vi "GaAs_GaP_wait_SL.vi"(2 "Debug Mode":bool, 3 "Elapsed Time(s)":dbl, 4 "State":enum16{"Edit", "Start", "Run", "End", "Idle"}(ring), 5 "Argument List In":string[](array[string])) -> (0 "Status Out":string, 1 "Argument List Out":string[](array[string]))   [LabVIEW 2011]
panel:
  out "tphase(s)":dbl[](array[numeric])
  out "nstep":dbl
  out "phase":i32
  out "done":bool
  in  "tP wait (s)":dbl
  in  "tP flow (s)":dbl
  in  "P flow (sccm)":dbl
  in  "nPeriods":dbl
  out "tTotal(s)":dbl
  out "tPeriod(s)":dbl
  in  "tAs wait (s)":dbl
  in  "tAs flow (s)":dbl
  in  "As flow (sccm)":dbl
  in  "Cancel":bool
  in  "OK":bool
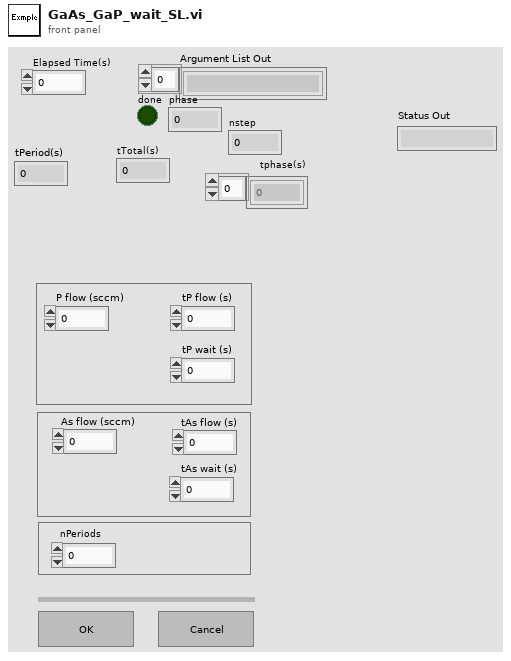
[diagram p1: front panel]
types:
  T1 = enum16{"Discrete", "Continuous", "Instantaneous"}
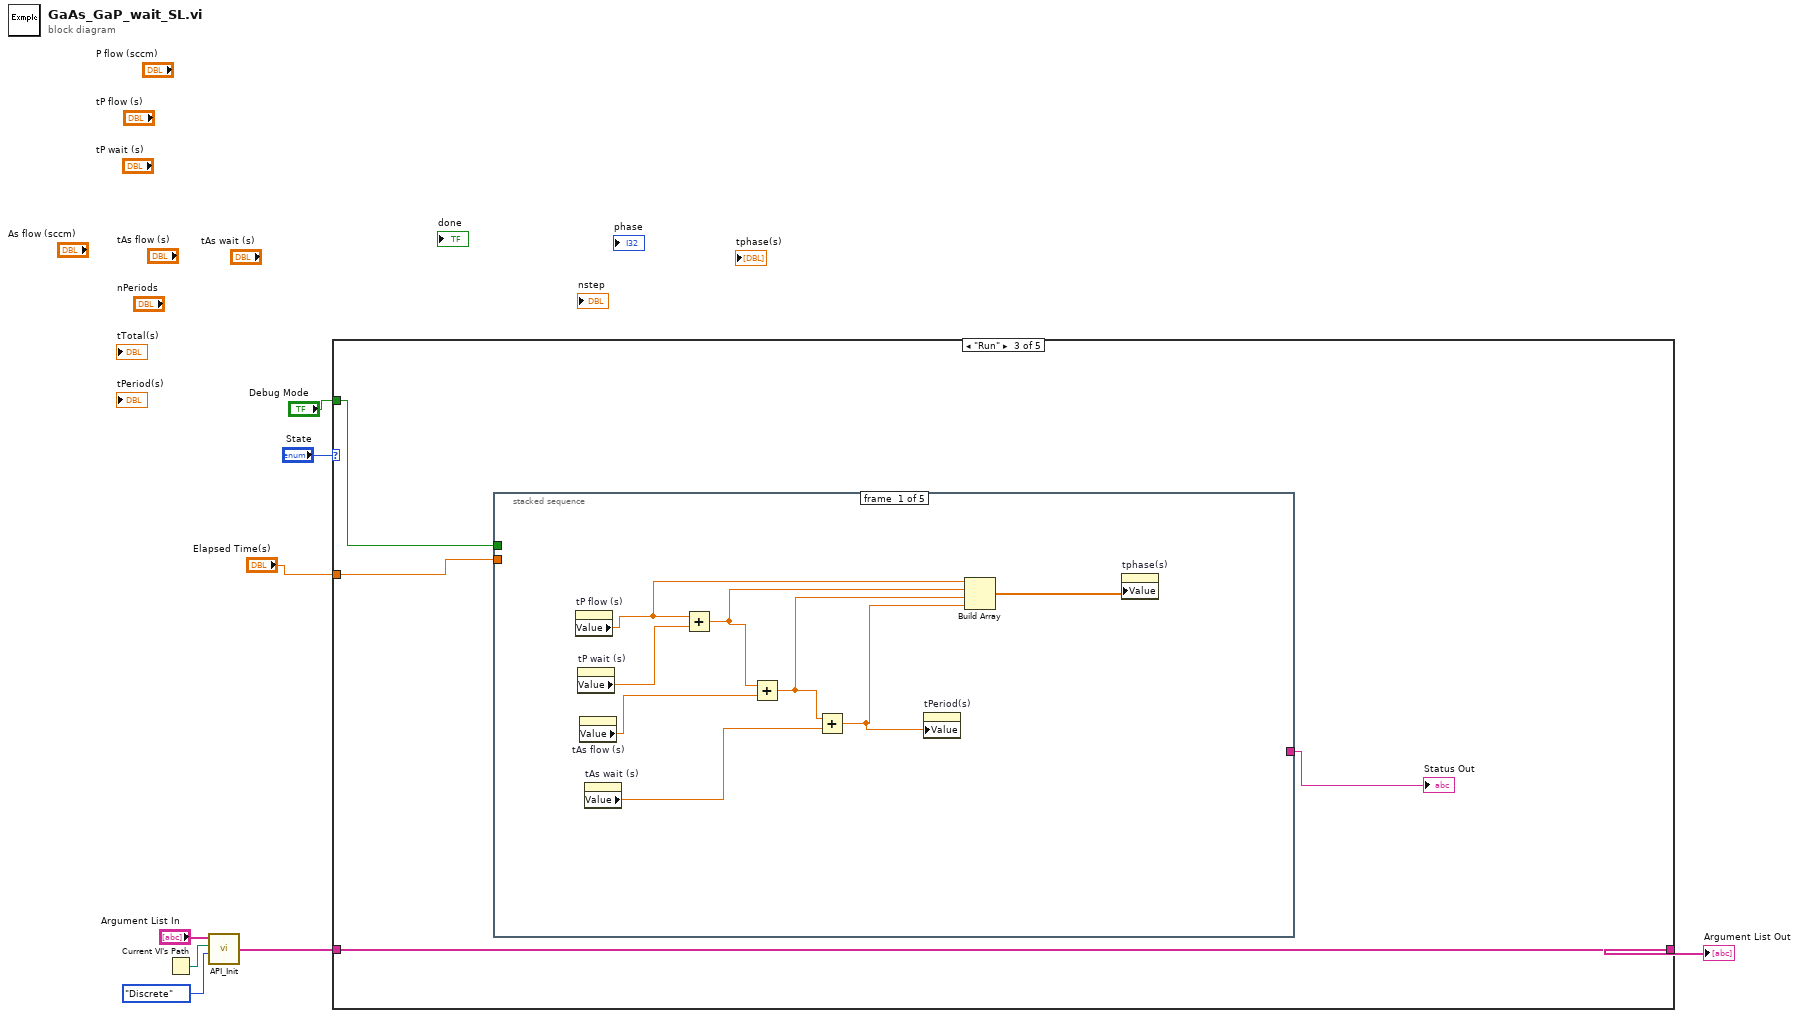
[diagram p0: block diagram]
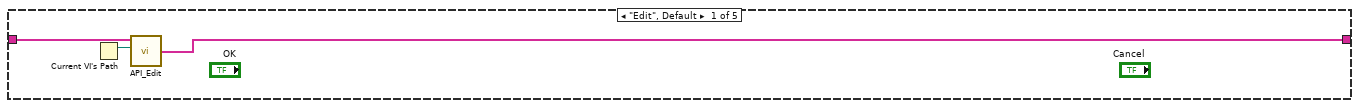
[diagram p2: hidden frame]
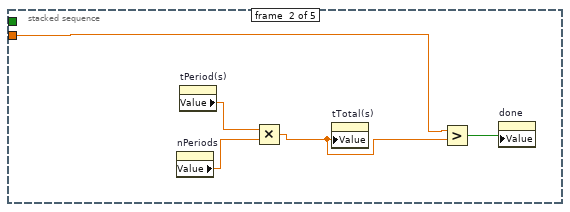
[diagram p4: hidden frame]
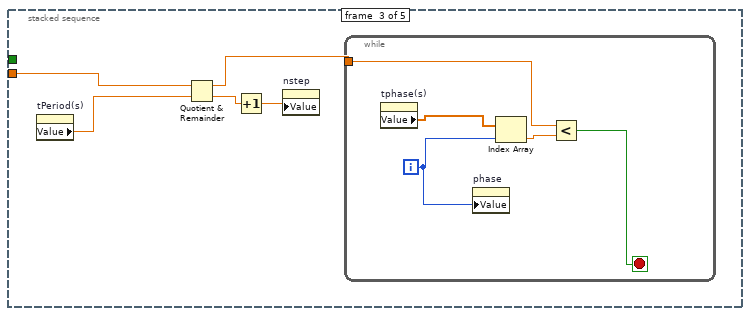
[diagram p5: hidden frame]
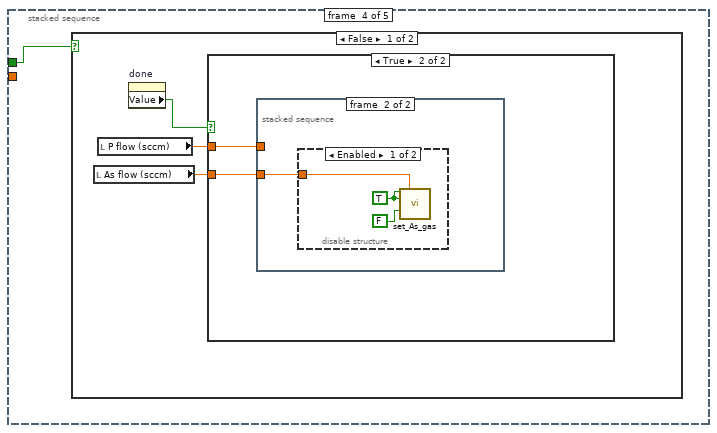
[diagram p6: hidden frame]
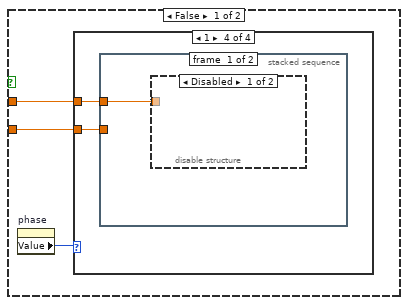
[diagram p7: hidden frame]
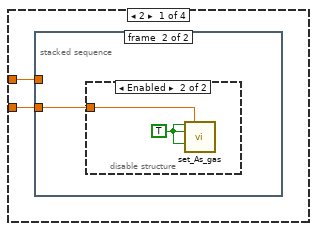
[diagram p8: hidden frame]
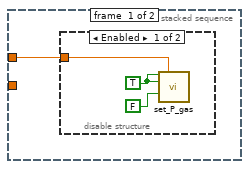
[diagram p9: hidden frame]
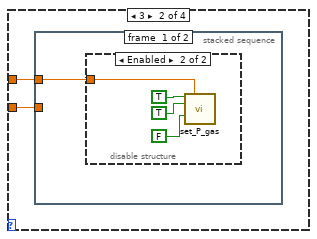
[diagram p12: hidden frame]
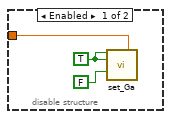
[diagram p15: hidden frame]
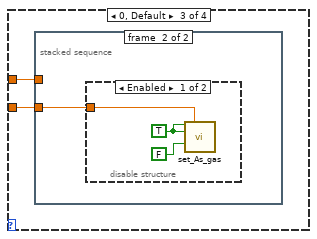
[diagram p16: hidden frame]
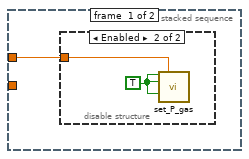
[diagram p17: hidden frame]
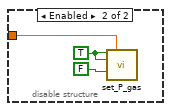
[diagram p20: hidden frame]
diagram:
  n1 = Current VI's Path() -> (path=w5:path)
  n2 = call "API_Init.vi"("API Mode"=T1."Discrete", "VI Path"=w5, "Argument List In"="Argument List In") -> ("Argument List Out"=w6:string[])  [unwired: 1 in]
  n3 = case shown="\"Run\"" "State" {
    tunnel: [w9 w12 w16 w127 w128] -> w2
    tunnel: w6 -> [w11 w12 w16 w127 w128]
    tunnel: "Debug Mode" -> [_ _ w14 _ _]
    tunnel: "Elapsed Time(s)" -> [_ _ w15 _ _]
    frame "Edit", Default {
      n4 = Current VI's Path() -> (path=w10:path)
      n5 = call "API_Edit.vi"("VI Path"=w10, "Argument List In"=w11) -> ("Argument List Out"=w9:string[])  [unwired: 2 in]
    }
    frame "Start" {
    }
    frame "Run" {
      n6 = stacked-sequence {
        tunnel: w15 -> [_ w27 w34 _ _]
        tunnel: w14 -> [_ _ _ w40 _]
        tunnel: [_ _ _ _ w96] -> w13
        frame #0 {
          n7 = property on="tP flow (s)" class="DigNum (strict)"() -> ("Value"=w23:dbl)  [unwired: 2 in, 2 out]
          n8 = property on="tP wait (s)" class="DigNum (strict)"() -> ("Value"=w24:dbl)  [unwired: 2 in, 2 out]
          n9 = property on="tAs flow (s)" class="DigNum (strict)"() -> ("Value"=w21:dbl)  [unwired: 2 in, 2 out]
          n10 = property on="tAs wait (s)" class="DigNum (strict)"() -> ("Value"=w20:dbl)  [unwired: 2 in, 2 out]
          n11 = Add(x=w23, y=w24) -> (x+y=w22:dbl)
          n12 = Add(x=w22, y=w21) -> (x+y=w19:dbl)
          n13 = Add(x=w19, y=w20) -> (x+y=w18:dbl)
          n14 = property on="tPeriod(s)" class="DigNum (strict)"("Value"=w18) -> ()  [unwired: 2 in, 2 out]
          n15 = Build Array(w23, w22, w19, w18) -> (w17:dbl[])
          n16 = property on="tphase(s)" class="Arr (strict)"("Value"=w17) -> ()  [unwired: 2 in, 2 out]
        }
        frame #1 {
          n17 = property on="nPeriods" class="DigNum (strict)"() -> ("Value"=w28:dbl)  [unwired: 2 in, 2 out]
          n18 = property on="tPeriod(s)" class="DigNum (strict)"() -> ("Value"=w29:dbl)  [unwired: 2 in, 2 out]
          n19 = Multiply(x=w29, y=w28) -> (x*y=w26:dbl)
          n20 = property on="tTotal(s)" class="DigNum (strict)"("Value"=w26) -> ()  [unwired: 2 in, 2 out]
          n21 = Greater?(x=w27, y=w26) -> (0:w25:bool)
          n22 = property on="done" class="Bool (strict)"("Value"=w25) -> ()  [unwired: 2 in, 2 out]
        }
        frame #2 {
          n23 = property on="tPeriod(s)" class="DigNum (strict)"() -> ("Value"=w33:dbl)  [unwired: 2 in, 2 out]
          n24 = Quotient & Remainder(x=w34, y=w33) -> (x-y*floor(x/y)=w32:dbl, floor(x/y)=w31:dbl)
          n25 = Increment(x=w31) -> (x+1=w30:dbl)
          n26 = property on="nstep" class="DigNum (strict)"("Value"=w30) -> ()  [unwired: 2 in, 2 out]
          n27 = while {
            tunnel: w32 -> [w38]
            i -> [w36]
            stop <- w35 stop-if-true
            n28 = property on="tphase(s)" class="Arr (strict)"() -> ("Value"=w39:dbl[])  [unwired: 2 in, 2 out]
            n29 = property on="phase" class="DigNum (strict)"("Value"=w36) -> ()  [unwired: 2 in, 2 out]
            n30 = Index Array(array=w39, index=w36) -> (element=w37:dbl)
            n31 = Less?(x=w38, y=w37) -> (x < y?=w35:bool)
          }
        }
        frame #3 {
          n32 = case shown="False" w40 {
            frame False {
              n33 = local read "As flow (sccm)"() -> (w43:dbl)
              n34 = local read "P flow (sccm)"() -> (w42:dbl)
              n35 = property on="done" class="Bool (strict)"() -> ("Value"=w41:bool)  [unwired: 2 in, 2 out]
              n36 = case shown="True" w41 {
                tunnel: w43 -> [w46 w86]
                tunnel: w42 -> [w45 w87]
                frame False {
                  n37 = property on="phase" class="DigNum (strict)"() -> ("Value"=w44:i32)  [unwired: 2 in, 2 out]
                  n38 = case shown="1" w44 {
                    tunnel: w45 -> [w48 w57 w68 w77]
                    tunnel: w46 -> [w47 w56 w67 w76]
                    frame 2 {
                      n39 = stacked-sequence {
                        tunnel: w48 -> [w49 _]
                        tunnel: w47 -> [_ w53]
                        frame #0 {
                          n40 = disable-structure shown="Enabled" {
                            disable-tunnel: w49 -> [w50 _]
                            frame Enabled {
                              w52 = TRUE ("Ga Active")
                              n41 = call "set_P_gas.vi"("P_Gas Active"=w52, "P_Gas Flow"=w50, "P_Gas In"=w52, "P_Gas Run"=FALSE ("Al Run")) -> ()  [unwired: 12 in]
                            }
                            frame Disabled {
                            }
                          }
                        }
                        frame #1 {
                          n42 = disable-structure shown="Enabled" {
                            disable-tunnel: w53 -> [_ w55]
                            frame Disabled {
                            }
                            frame Enabled {
                              w54 = TRUE ("Ga Active")
                              n43 = call "set_As_gas.vi"("As_Gas Active"=w54, "As_Gas Flow"=w55, "As_Gas In"=w54, "As_Gas Run"=w54) -> ()  [unwired: 12 in]
                            }
                          }
                        }
                      }
                    }
                    frame 3 {
                      n44 = stacked-sequence {
                        tunnel: w57 -> [w58 _]
                        tunnel: w56 -> [_ w63]
                        frame #0 {
                          n45 = disable-structure shown="Enabled" {
                            disable-tunnel: w58 -> [_ w59]
                            frame Disabled {
                            }
                            frame Enabled {
                              n46 = call "set_P_gas.vi"("P_Gas Active"=TRUE ("Al Active"), "P_Gas Flow"=w59, "P_Gas In"=TRUE ("Al Bubbler"), "P_Gas Run"=FALSE ("Al Run")) -> ()  [unwired: 12 in]
                            }
                          }
                        }
                        frame #1 {
                          n47 = disable-structure shown="Disabled" {
                            disable-tunnel: w63 -> [w64 _]
                            frame Enabled {
                              w65 = TRUE ("Ga Active")
                              n48 = call "set_Ga.vi"("Ga Active"=w65, "Ga Flow 1"=w64, "Ga Bubbler"=w65, "Ga Run"=FALSE) -> ()  [unwired: 4 in, 8 out]
                            }
                            frame Disabled {
                            }
                          }
                        }
                      }
                    }
                    frame 0, Default {
                      n49 = stacked-sequence {
                        tunnel: w68 -> [w69 _]
                        tunnel: w67 -> [_ w72]
                        frame #0 {
                          n50 = disable-structure shown="Enabled" {
                            disable-tunnel: w69 -> [_ w71]
                            frame Disabled {
                            }
                            frame Enabled {
                              w70 = TRUE ("Al Active")
                              n51 = call "set_P_gas.vi"("P_Gas Active"=w70, "P_Gas Flow"=w71, "P_Gas In"=w70, "P_Gas Run"=w70) -> ()  [unwired: 12 in]
                            }
                          }
                        }
                        frame #1 {
                          n52 = disable-structure shown="Enabled" {
                            disable-tunnel: w72 -> [w73 _]
                            frame Enabled {
                              w74 = TRUE ("Ga Active")
                              n53 = call "set_As_gas.vi"("As_Gas Active"=w74, "As_Gas Flow"=w73, "As_Gas In"=w74, "As_Gas Run"=FALSE ("Ga Run")) -> ()  [unwired: 12 in]
                            }
                            frame Disabled {
                            }
                          }
                        }
                      }
                    }
                    frame 1 {
                      n54 = stacked-sequence {
                        tunnel: w76 -> [_ w82]
                        tunnel: w77 -> [w78 _]
                        frame #0 {
                          n55 = disable-structure shown="Disabled" {
                            disable-tunnel: w78 -> [_ w80]
                            frame Disabled {
                            }
                            frame Enabled {
                              w79 = TRUE ("Al Bubbler")
                              n56 = call "set_P_gas.vi"("P_Gas Active"=w79, "P_Gas Flow"=w80, "P_Gas In"=w79, "P_Gas Run"=FALSE ("Al Run")) -> ()  [unwired: 12 in]
                            }
                          }
                        }
                        frame #1 {
                          n57 = disable-structure shown="Disabled" {
                            disable-tunnel: w82 -> [w83 _]
                            frame Enabled {
                              w84 = TRUE ("Ga Active")
                              n58 = call "set_As_gas.vi"("As_Gas Active"=w84, "As_Gas Flow"=w83, "As_Gas In"=w84, "As_Gas Run"=FALSE ("Ga Run")) -> ()  [unwired: 12 in]
                            }
                            frame Disabled {
                            }
                          }
                        }
                      }
                    }
                  }
                }
                frame True {
                  n59 = stacked-sequence {
                    tunnel: w87 -> [w88 _]
                    tunnel: w86 -> [_ w92]
                    frame #0 {
                      n60 = disable-structure shown="Enabled" {
                        disable-tunnel: w88 -> [_ w91]
                        frame Disabled {
                        }
                        frame Enabled {
                          w90 = TRUE ("Al Active")
                          n61 = call "set_Al.vi"("Aluminum Flow"=w91, "Al Run"=FALSE, "Al Bubbler"=w90, "Al Active"=w90) -> ()  [unwired: 6 in]
                        }
                      }
                    }
                    frame #1 {
                      n62 = disable-structure shown="Enabled" {
                        disable-tunnel: w92 -> [w93 _]
                        frame Enabled {
                          w94 = TRUE ("Ga Active")
                          n63 = call "set_As_gas.vi"("As_Gas Active"=w94, "As_Gas Flow"=w93, "As_Gas In"=w94, "As_Gas Run"=FALSE ("Ga Run")) -> ()  [unwired: 12 in]
                        }
                        frame Disabled {
                        }
                      }
                    }
                  }
                }
              }
            }
            frame True {
            }
          }
        }
        frame #4 {
          n64 = property on="done" class="Bool (strict)"() -> ("Value"=w97:bool)  [unwired: 2 in, 2 out]
          n65 = case shown="True" w97 {
            tunnel: [w98 w126] -> w96
            frame False {
              n66 = property on="phase" class="DigNum (strict)"() -> ("Value"=w105:i32)  [unwired: 2 in, 2 out]
              n67 = case shown="0, Default" w105 {
                tunnel: [w108 "wait (Ga)" w115 "wait (Al)"] -> w104
                frame 2 {
                  n68 = local read "As flow (sccm)"() -> (w107:dbl)
                  n69 = Format Into String(format string="%4.2f", w107) -> (resulting string=w111:string)  [unwired: 2 in, 1 out]
                  n70 = Concatenate Strings("Ga(" ("string"), w111, "sccm)" ("string")) -> (w108:string)
                }
                frame 3 {
                }
                frame 0, Default {
                  n71 = local read "P flow (sccm)"() -> (w114:dbl)
                  n72 = Format Into String(format string="%4.1f", w114) -> (resulting string=w117:string)  [unwired: 2 in, 1 out]
                  n73 = Concatenate Strings("Al(" ("string"), w117, "sccm)" ("string")) -> (w115:string)
                }
                frame 1 {
                }
              }
              n74 = property on="nstep" class="DigNum (strict)"() -> ("Value"=w106:dbl)  [unwired: 2 in, 2 out]
              n75 = Format Into String(format string="%3.0f", w106) -> (resulting string=w101:string)  [unwired: 2 in, 1 out]
              n76 = Concatenate Strings("Period " ("string"), w101) -> (w99:string)
              n77 = Concatenate Strings(w99, ", " ("string"), w104) -> (w98:string)
            }
            frame True {
              n78 = property on="nPeriods" class="DigNum (strict)"() -> ("Value"=w121:dbl)  [unwired: 2 in, 2 out]
              n79 = Format Into String(format string="%3.0f", w121) -> (resulting string=w122:string)  [unwired: 2 in, 1 out]
              n80 = Concatenate Strings("done after", w122, " periods" ("string")) -> (w126:string)
            }
          }
        }
      }
      "Status Out" <- w13
    }
    frame "End" {
    }
    frame "Idle" {
    }
  }
  "Argument List Out" <- w2
